vi "Modify JSON-Example.vi"() -> ()   [LabVIEW 2015]
uses:
  <vilib>/addons/_JKI.lib/Serialization/JSON/JKI JSON Serialization.lvlib
panel:
  out "Functionality Error Message out":string
  out "Functionality Applied":T1(ring)
  in  "error in (no error)":errorcluster
  in  "JSON Hierarchy":string="$.2DArray[2]"
  in  "Functionality":T1(ring)=enum."Replace"
  out "JSON String":string
  out "Syntax Error Message out":string
  out "error out":errorcluster
  in  "Input String":string="{\n\"String1\": \"string1\",\n\"String2\": \"string2\",\n\"U321\": 4324,\n\"U322\": 6546456,\n\"boolean1\": true,\n\"boolean2\": false,\n\"double1\": 1.0,\n\"double2\": 323.43432,\n\"double3\": -31231.0,\n\"SignedInteger1\": -12,\n\"Cluster1\": {\n\"String1\": \"string1\",\n\"num1\": 12,\n\"boolean\": true\n},\n\"Cluster2\": {\n\"String1\": \"string1\",\n\"num1\": 12,\n\"boolean\": true,\n\"NestedCluster1\": {\n\"String1\": \"string1\",\n\"num1\": 12,\n\"boolean\": true,\n\"NestedCluster11\": {\n\"String1\": \"string1\",\n\"num1\": 12,\n\"boolean\": true\n}\n}\n},\n\"ArrayOfString\": [\"abc\",\"def\",\"ghi\",\"jkl\",\"mnop\",\"qrs\",\"twu\",\"vxy\",\"z\"],\n\"ArrayOfBoolean\": [true,false,true,true,false],\n\"ArrayOfU64\": [32,43,54],\n\"ArrayOfI32\": [-32,43,54,-12],\n\"ArrayOfDouble\": [2.0,4.0,5.0],\n\"ArrayOfClusters1\": [\n{\n\"String1\": \"string 1.1\",\n\"num1\": 12,\n\"boolean\": true\n},\n{\n\"String1\": \"string 1.2\",\n\"num1\": 12,\n\"boolean\": true\n},\n{\n\"String1\": \"string 1.3\",\n\"num1\": 13,\n\"boolean\": true\n},\n{\n\"String1\": \"string 4\",\n\"num1\": 14,\n\"boolean\": true\n}\n],\n\"NestedClusters\": {\n\"Cluster1\": {\n\"Name\": \"test1\",\n\"number\": 1.0,\n\"Cluster2\": {\n\"Name\": \"test11\",\n\"Number\": 1.1,\n\"Cluster3\": {\n\"Name\": \"test111\",\n\"Number\": 1.2,\n\"Cluster4\": {\n\"Name\": \"test1111\",\n\"Number\": 1.3,\n\"Cluster5\": {\n\"Name\": \"test11111\",\n\"Number\":  1.4\n}\n}\n}\n}\n}\n},\n\"ArrayOfClusters2\": [\n{\n\"String1\": \"string 1.1\",\n\"num1\": 12,\n\"boolean\": true,\n\"ArrayOfClusters\": [\n{\n\"String1\": \"string 2.1\",\n\"num1\": 12,\n\"boolean\": true\n},\n{\n\"String1\": \"string 2.2\",\n\"num1\": 12,\n\"boolean\": true\n},\n{\n\"String1\": \"string 2.3\",\n\"num1\": 13,\n\"boolean\": true\n},\n{\n\"String1\": \"string 2.4\",\n\"num1\": 14,\n\"boolean\": true\n}\n]\n},\n{\n\"String1\": \"string 1.1\",\n\"num1\": 12,\n\"boolean\": true,\n\"ArrayOfClusters\": [\n{\n\"String1\": \"string 3.1\",\n\"num1\": 12,\n\"boolean\": true\n},\n{\n\"String1\": \"string 3.2\",\n\"num1\": 12,\n\"boolean\": true\n},\n{\n\"String1\": \"string 3.3\",\n\"num1\": 13,\n\"boolean\": true\n},\n{\n\"String1\": \"string 3.4\",\n\"num1\": 14,\n\"boolean\": true\n}\n]\n},\n{\n\"String1\": \"string 1.1\",\n\"num1\": 12,\n\"boolean\": true,\n\"ArrayOfClusters\": [\n{\n\"String1\": \"string 4.1\",\n\"num1\": 12,\n\"boolean\": true\n},\n{\n\"String1\": \"string 4.2\",\n\"num1\": 12,\n\"boolean\": true\n},\n{\n\"String1\": \"string 4.3\",\n\"num1\": 13,\n\"boolean\": true\n},\n{\n\"String1\": \"string 4.4\",\n\"num1\": 14,\n\"boolean\": true\n}\n]\n}\n],\n\"2DArray\": [\n[1,2,3],\n[3,4,5],\n[6,7,8]\n]\n}\n\n\n\n"
  # "Press Ctrl+R to run the current \nprogram.\nThe following can be changed based\nupon the requirement :\n1. JSON file path\n2. PathList (To Replace / Insert / Append the data)\n3. Cluster1 (based upon the data which needs to be \nReplace/Inserted/Appended)"
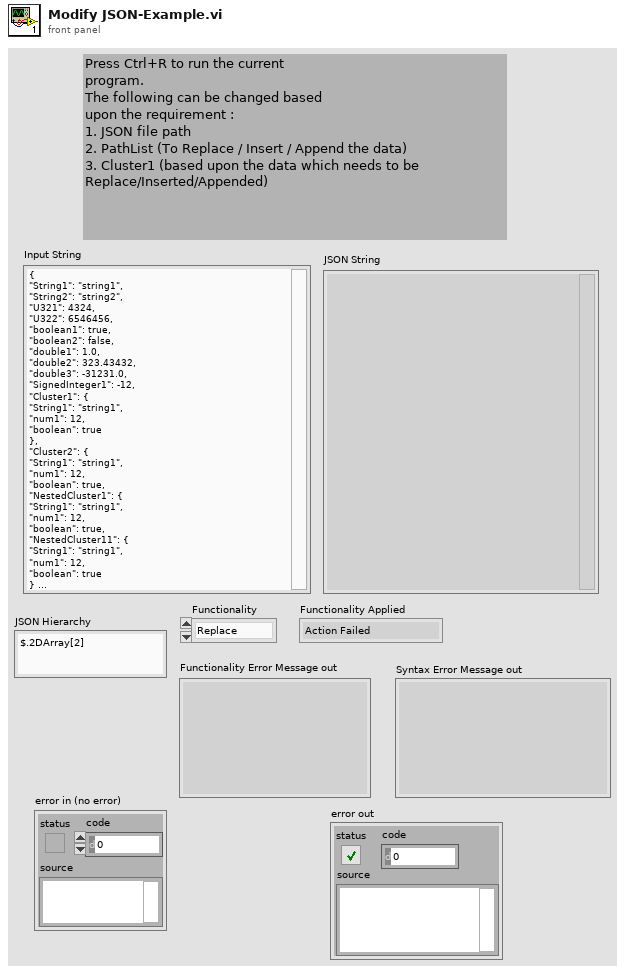
[diagram p1: front panel]
types:
  T1 = enum16{"Action Failed", "Append", "Insert", "Replace"}
  T2 = cluster{"num1":i32, "String1":string, "boolean":bool}
  T3 = cluster{"String1":string, "num1":i32, "boolean":bool}
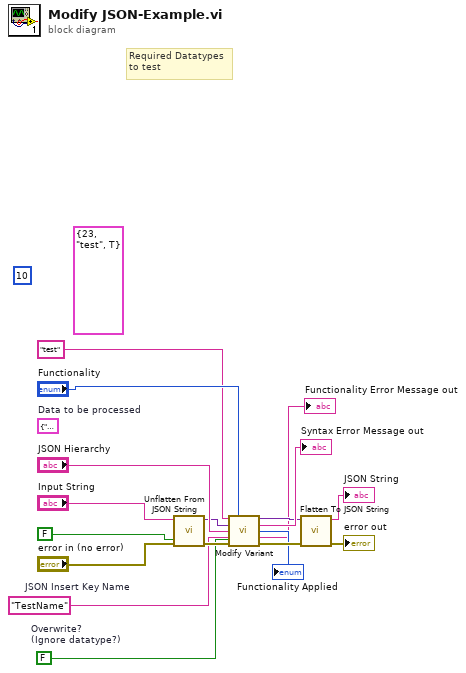
[diagram p0: block diagram]
diagram:
  (unwired) T2 {"num1"=23, "String1"="test", "boolean"=TRUE}
  (unwired) u64 10
  (unwired) T3 {"String1"="Test", "num1"=289, "boolean"=TRUE}  # Data to be processed
  w5 = "TestName"  # JSON Insert Key Name
  w9 = FALSE  # Overwrite? (Ignore datatype?)
  # "Required Datatypes\nto test"
  n1 = call <vilib>:"Unflatten From JSON String.vi"("Nulls as Defaults (F)"=FALSE, "error in (no error)"="error in (no error)", "JSON String"="Input String") -> ("error out"=w16:errorcluster, "Variant"=w7:variant)  [unwired: 7 in]
  n2 = call "Modify Variant.vi"("New element in"="test", "Functionality"="Functionality", "Parent variant in"=w7, "JSON query path"="JSON Hierarchy", "JSON New Element Key Name"=w5, "error in (no error)"=w16, "Overwrite\n(Ignore datatype?)"=w9) -> ("VCluster out"=w14:variant, "Syntax Error Message out"=→"Syntax Error Message out":string, "Functionality Applied"=→"Functionality Applied":T1, "Functionality Error Message out"=→"Functionality Error Message out":string, "error out"=w15:errorcluster)  [unwired: 4 in]
  n3 = call <vilib>:"Flatten To JSON String.vi"("error in (no error)"=w15, "Variant"=w14) -> ("error out"=→"error out":errorcluster, "JSON String"=→"JSON String":string)  [unwired: 8 in]
